vi "Creat_DIR.vi"(11 "path":path caption="路径") -> (3 "created path":path)   [LabVIEW 2020]
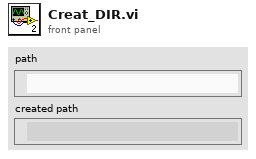
[diagram p1: front panel]
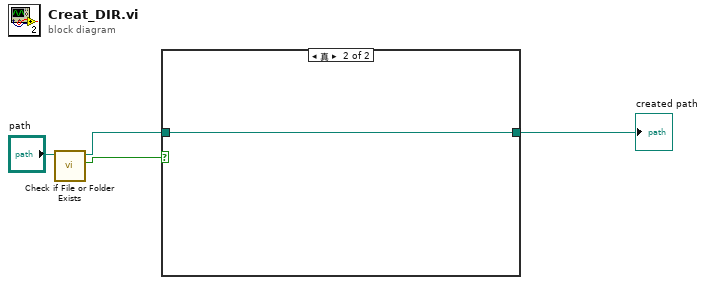
[diagram p0: block diagram]
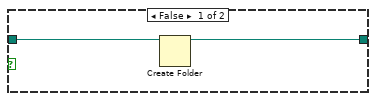
[diagram p2: hidden frame]
diagram:
  n1 = call <vilib>:"Check if File or Folder Exists.vi"("path"="path") -> ("file or folder exists?"=w3:bool, "dup path"=w2:path)  [unwired: 8 in, 1 out]
  n2 = case shown="真" w3 {
    tunnel: w2 -> [w6 w7]
    tunnel: [w5 w7] -> w1
    frame False {
      n3 = Create Folder(path (use dialog)=w6) -> (created path=w5:path)  [unwired: 2 in, 2 out]
    }
    frame True {
    }
  }
  "created path" <- w1
